vi "locate engine by value.vi"(8 "error in":errorcluster, 11 "Node":refnum<class "NISE_CEF_Node.lvclass">) -> (0 "error out":errorcluster, 3 "engine":refnum<data-value>)   [LabVIEW 2013, in "PL Framework Configuration Tool.lvlib" / "module editor node.lvclass"]
uses:
  module editor node.lvclass
  Engine Parent/Engine Parent Editor Node.lvclass
  <vilib>/NI/Configuration Framework/Node/NISE_CEF_Node.lvclass
  <vilib>/NI/Configuration Framework/Node/NISE_CEF_Node.lvclass/NISE_CEF_Node.ctl
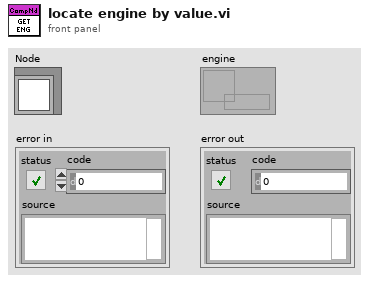
[diagram p1: front panel]
types:
  T1 = typedef "NISE_CEF_Node.lvclass/NodeRef.ctl" = refnum<data-value>
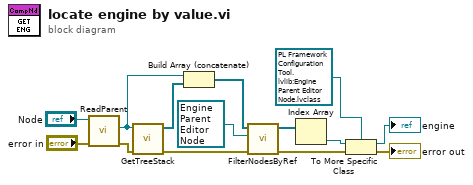
[diagram p0: block diagram]
diagram:
  n1 = call <vilib>:"ReadParent.vi"("error in"="error in", "node in"="Node") -> ("error out"=w1:errorcluster, "parent"=w4:T1)  [unwired: 7 in, 1 out]
  n2 = call <vilib>:"GetTreeStack.vi"("error in"=w1, "node in"=w4) -> ("error out"=w11:errorcluster, "parents"=w12:refnum<data-value>[])  [unwired: 8 in]
  n3 = Build Array (concatenate)(w4, w12) -> (w5:T1[])
  n4 = call <vilib>:"FilterNodesByRef.vi"("error in"=w11, "NISE_CEF_Node"=refnum<class "Engine Parent Editor Node.lvclass"> refnum ("PL Framework Configuration Tool.lvlib:Engine Parent Editor Node.lvclass"), "nodes"=w5) -> ("error out"=w8:errorcluster, "filtered nodes"=w9:refnum<data-value>[])  [unwired: 7 in]
  n5 = Index Array(array=w9) -> (element=w7:refnum<data-value>)  [unwired: 1 in]
  n6 = To More Specific Class(target class=refnum<data-value> refnum, reference=w7, error in=w8) -> (specific class reference=→"engine":refnum<data-value>, error out=→"error out":errorcluster)
